vi "Read 2 measurement Channels Osciloscope.vi"(8 "error in (no error)":errorcluster, 10 "Read 2 channels In":T1={"Channel 1 (1: Channel 1)"=1, "Channel 2 (2: Channel 2)"=2, "Measurement Type (0: Phase)"=0} {"Measurement Type (0: Phase)" items=["Phase", "Delay", "DelayRR", "DelayRF", "DelayFR", "DelayFF"]; "Channel 2 (2: Channel 2)" items=["Channel 1"=1, "Channel 2"=2, "Channel 3"=3, "Channel 4"=4]; "Channel 1 (1: Channel 1)" items=["Channel 1"=1, "Channel 2"=2, "Channel 3"=3, "Channel 4"=4]}, 11 "Tektronicks in":refnum<class "Tektronicks.lvclass">) -> (0 "error out":errorcluster, 2 "Read 2 channels Out":T2, 3 "Tektronicks out":refnum<class "Tektronicks.lvclass">)   [LabVIEW 2020, in "Tektronicks.lvclass"]
uses:
  Tektronicks.lvclass
  TypeDefs/Read2ChannlesOut.ctl
  TypeDefs/Read2channelsIn--cluster.ctl
  Tektronicks.lvclass/Tektronicks.ctl
  <instrlib>/Tektronix TDS 200 1000 2000 Series/Tektronix TDS 200 1000 2000 Series.lvlib
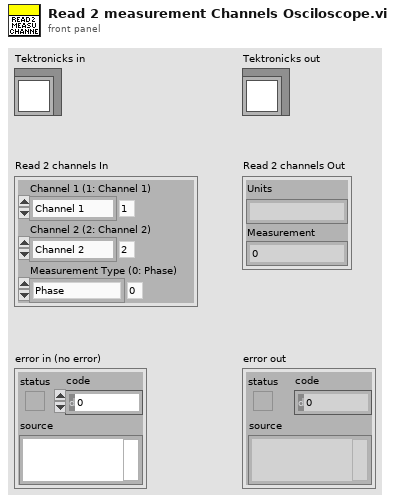
[diagram p1: front panel]
types:
  T1 = typedef "Read2channelsIn--cluster.ctl" = cluster{"Channel 1 (1: Channel 1)":i32, "Channel 2 (2: Channel 2)":i32, "Measurement Type (0: Phase)":i32}
  T2 = typedef "Read2ChannlesOut.ctl" = cluster{"Units":string, "Measurement":dbl}
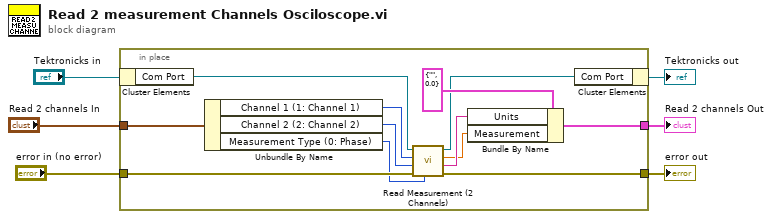
[diagram p0: block diagram]
diagram:
  n1 = in-place {
    in-place-border: "error in (no error)" -> [w18]
    in-place-border: [w17] -> w3
    in-place-border: "Read 2 channels In" -> [w16]
    in-place-border: [w12] -> w1
    n2 = in-place-cluster #1("Tektronicks in") -> ("Com Port"=w7:refnum<visa-resource-name>)
    n3 = Unbundle By Name(w16) -> ("Channel 1 (1: Channel 1)"=w15:i32, "Channel 2 (2: Channel 2)"=w14:i32, "Measurement Type (0: Phase)"=w13:i32)
    n4 = call <instrlib>:"Read Measurement (2 Channels).vi"("Measurement Type (0: Phase)"=w13, "error in (no error)"=w18, "Channel 2 (2: Channel 2)"=w14, "Channel 1 (1: Channel 1)"=w15, "VISA resource name"=w7) -> ("error out"=w17:errorcluster, "Units"=w10:string, "Measurement"=w9:dbl, "VISA resource name out"=w8:refnum<visa-resource-name>)  [unwired: 3 in]
    n5 = Bundle By Name(cluster=T2 {"Units"="", "Measurement"=0.0} ("Read 2 channels Out"), "Units"=w10, "Measurement"=w9) -> (w12:T2)
    n6 = in-place-cluster #1("Com Port"=w8) -> (→"Tektronicks out":refnum<class "Tektronicks.lvclass">)
  }
  "error out" <- w3
  "Read 2 channels Out" <- w1
